vi "matlabview.vi"() -> ()   [LabVIEW 2023]
panel:
  out "Theta_graden":dbl
  in  "source file path":path
  in  "Dist":dbl
  out "error out":errorcluster
  in  "error in (no error)":errorcluster
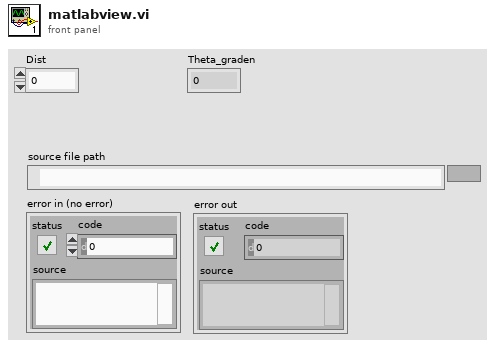
[diagram p1: front panel]
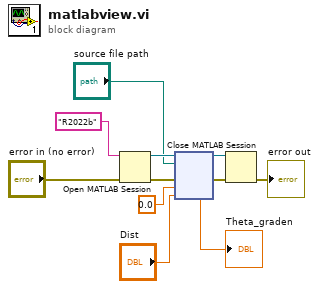
[diagram p0: block diagram]
diagram:
  n1 = Open MATLAB Session(0:"R2022b" ("release name"), 3:"error in (no error)") -> (8:w11:refnum<k37>, 11:w6:errorcluster)
  n2 = node(w11, "source file path", w6, 0.0, "Dist") -> (w10:refnum<k37>, w4:errorcluster, →"Theta_graden":dbl)  [unwired: 2 in, 2 out]
  n3 = Close MATLAB Session(0:w10, 3:w4) -> (11:→"error out":errorcluster)
